vi "Dashboard Main.vi"() -> ()   [LabVIEW 2018]
uses:
  <vilib>/Utility/miscctls.llb/LVRowAndColumnTypeDef.ctl
  <vilib>/event_ctls.llb/eventvkey.ctl
  <vilib>/Rock Robotics/Network Tables/NT Read Boolean.vi
  <vilib>/Rock Robotics/WPI/Dashboard/WPI_DashboardLogging Global.vi
panel:
  in  "Camera Settings Right":T1={"Frame Rate"=30, "Compression"=30, "Size"=1, "DB Camera Config"=FALSE} {"Frame Rate" scale=1.0..30.0; "Compression" scale=100.0..-1.0; "Size" items=["640x480", "320x240", "160x120"]}
  in  "Camera Name Right":string(combo)="No Camera Selection"
  out "Camera Perf":string
  in  "Camera Settings":T1={"Frame Rate"=30, "Compression"=30, "Size"=1, "DB Camera Config"=FALSE} {"Frame Rate" scale=1.0..30.0; "Compression" scale=100.0..-1.0; "Size" items=["640x480", "320x240", "160x120"]}
  in  "TCP":refnum<k5>
  in  "Rec Mode":enum32{"Stop", "Record", "Playback"}(radio)
  out "Robot IP":string
  out "Image Message":string="Timeout in Camera Communications"
  in  "Dashboard Tab":T2(tab)
  out "Total":bool
  out "Total":dbl(slide) scale=0.0..150.0
  out "Intake":bool
  out "Intake":dbl(slide) scale=0.0..30.0
  out "B2":bool
  out "B1":bool
  out "B2":dbl(slide) scale=0.0..40.0
  out "B1":dbl(slide) scale=0.0..40.0
  out "EL2":bool
  out "EL1":bool
  out "EL2":dbl(slide) scale=0.0..40.0
  out "EL1":dbl(slide) scale=0.0..40.0
  out "BR":bool
  out "BL":bool
  out "FR":bool
  out "FL":bool
  out "BR":dbl(slide) scale=0.0..40.0
  out "BL":dbl(slide) scale=0.0..40.0
  out "FR":dbl(slide) scale=0.0..40.0
  out "FL":dbl(slide) scale=0.0..40.0
  in  "Select Auto":string(combo)="Select Autonomous ..."
  out "NT Connection":bool
  out "Gyro":dbl(knob) scale=0.0..360.0
  out "JS1 Z":dbl(slide) scale=-1.0..1.0 scale format="%#_2e"
  out "JS1 Graph":cluster{"X":dbl, "Y":dbl}[](graph)
  out "JS1 Buttons":T3
  out "JS2 Z":dbl(slide) scale=-1.0..1.0 scale format="%#_2e"
  out "JS2 Graph":cluster{"X":dbl, "Y":dbl}[](graph)
  out "JS2 Buttons":T3
  out "Mode":T4(ring)=enum."Auto Disabled"
  out "Right Camera Perf":cluster{"Bandwidth (Mbps)":dbl, "FPS":dbl}
  out "Camera Image Right":T5(plugin-control)
  in  "DB/String 9":string
  in  "DB/String 8":string
  in  "DB/String 7":string
  in  "DB/String 6":string
  in  "DB/String 5":string
  in  "DB/String 4":string
  in  "DB/String 3":string
  in  "DB/String 2":string
  in  "DB/String 1":string
  in  "DB/String 0":string
  in  "DB/Slider 0":dbl(slide) scale=0.0..5.0
  in  "DB/Slider 1":dbl(slide) scale=0.0..5.0
  in  "DB/Slider 2":dbl(slide) scale=0.0..5.0
  in  "DB/Slider 3":dbl(slide) scale=0.0..5.0
  out "DB/LED 3":bool
  out "DB/LED 2":bool
  out "DB/LED 1":bool
  out "DB/LED 0":bool
  in  "DB/Button 3":bool
  in  "DB/Button 2":bool
  in  "DB/Button 1":bool
  in  "DB/Button 0":bool caption="New Name"
  in  "Test Slider":dbl(slide) scale=0.0..100.0 scale format="%#_3g"
  in  "On/Off":bool caption="Solenoid"
  in  "Test Name":u16(ring) items=["Select the test to run..."]
  in  "Test Tree":string(tree)
  in  "Motor":cluster{"Value":dbl, "Enable":bool} {"Value" scale=-1.0..1.0 scale format="%#_3g"}
  out "Progress":T6 {"Test Progress" scale=0.0..100.0}
  in  "Rev/Fwd":cluster{"Forward":bool, "Reverse":bool}
  in  "Test Ring":u16(ring) items=["Monochrome", "Color"]
  out "Cmd Status":string
  in  "Execute Command":bool
  in  "Command Params":string[][](table)
  in  "Command Selection":i32(listbox)
  in  "CheckList":i32(listbox)
  out "Tree":string(tree)
  out "Camera Image":T5(plugin-control)
  out "Background":bool
  in  "Camera Name":string(combo)="No Camera Selection"
  # "HW"
  # "HW"
  # "Joysticks"
  # "Drive Motors"
  # "Elevator"
  # "Four Bar"
  # "Intake"
  # "Total"
  # "This tab is a great place for autonomous settings and robot-specific values.\nPlace controls and indicators inside this tab and match name to\nDashboard Variables on robot. You can also delete this comment."
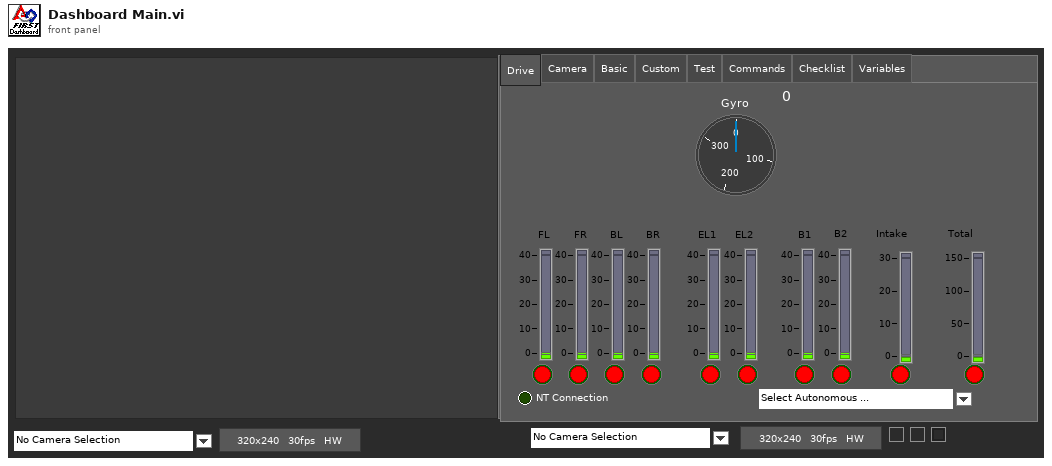
[diagram p1: front panel]
types:
  T1 = cluster{"Frame Rate":i32, "Compression":i32, "Size":u16, "DB Camera Config":bool}
  T2 = enum32{"Drive", "Camera", "Basic", "Custom", "Test", "Commands", "Checklist", "Variables"}
  T3 = cluster{bool, bool, bool, bool, bool, bool, bool, bool, bool, bool, bool, bool}
  T4 = enum8{"Tele-Op Disabled", "Tele-Op Enabled", "Auto Disabled", "Auto Enabled", "Test Disabled", "Test Enabled", "Disconnected", "No Code", "E-Stop"}
  T5 = typedef "IMAQ Image.ctl" = refnum<image>
  T6 = cluster{"Test Progress":u8, "Test Progress Text":string}
  T7 = cluster{"Save Path":path, "Interval (s)":dbl, "Keep":i32}
  T8 = typedef "Image Type" = u32
  T9 = cluster{"IDs":cluster{"RPC field ID":u16, "Unique ID":u16}, "String":string}
  T10 = cluster{"Error Strings":string, "Disable Counts":cluster{u16, u16}, "Rail Faults":cluster{u16, u16, u16}, "Robot IP":string, "DB Mode":u8, "Event Info":cluster{"Name":string, "Type":u8, "Number":u16, "Replay":u8}}
  T11 = cluster{"Storage":cluster{"Disk Free":u64, "RAM Block":u32, "RAM free":u32}, "CPU Utilization":cluster{"CPU % ISR":sgl, "CPU % Time Crit":sgl, "CPU % Timed Str":sgl, "CPU % High":sgl, "CPU % Above":sgl, "CPU % Normal":sgl, "CPU % Low":sgl}, "CAN":cluster{"% Bus Utilization":sgl, "Bus Off Cnt":u32, "TX_FIFO Full Cnt":u32, "Receive Error Cnt":u8, "Transmit Error Cnt":u8}, "HID":cluster{"HID Outputs":u32, "Rumble Low":u16, "Rumble High":u16}[]}
  T12 = cluster{"Status bits":cluster{"Test Mode":bool, "Autonomous":bool, "Enabled":bool, "Code Start":bool, "Brownout":bool, "Reserved 2":bool, "Reserved 3":bool, "E-Stop":bool}, "Code Trace":cluster{"Disabled":bool, "TeleOp":bool, "Auto":bool, "Test":bool}, "Controller Type":enum16{"unknown", "cRIO", "roboRio"}, "Code?":enum16{"unknown", "noCode", "code"}, "Battery V":dbl}
  T13 = cluster{"Control Bits":cluster{"TestMode":bool, "Autonomous":bool, "Enabled":bool, "FMS Present":bool, bool, bool, bool, "E-Stop":bool}, "Team Station ":u8, "Countdown":sgl, "Joystick Values":cluster{"Axes":dbl[], "Buttons":bool[], "POVs":i16[]}[]}
  T14 = cluster{"Axes":dbl[], "Buttons":bool[], "POVs":i16[]}[]
  T15 = cluster{"Axes":dbl[], "Buttons":bool[], "POVs":i16[]}
  T16 = cluster{"Buttons[0]":bool, "Buttons[1]":bool, "Buttons[2]":bool, "Buttons[3]":bool, "Buttons[4]":bool, "Buttons[5]":bool, "Buttons[6]":bool, "Buttons[7]":bool, "Buttons[8]":bool, "Buttons[9]":bool, "Buttons[10]":bool, "Buttons[11]":bool}
  T17 = cluster{"Camera Image":refnum<vi>, "Dashboard Tab":refnum<vi>, "Background":refnum<vi>, "Rec Mode":refnum<vi>, "Test Slider":refnum<vi>, "On/Off ":refnum<vi>, "Test Ring":refnum<vi>, "Rev/Fwd":refnum<vi>, "Test Name":refnum<vi>, "Motor":refnum<vi>, "Progress":refnum<vi>, "CheckList":refnum<vi>, "Tree":refnum<vi>, "Test Tree":refnum<vi>, "Command Params":refnum<vi>, "Command Selection":refnum<vi>, "Execute Command":refnum<vi>, "Cmd Status":refnum<vi>, "Camera Settings":refnum<vi>, "Camera Name":refnum<vi>, "Camera Perf":refnum<vi>, "Camera Settings Right":refnum<vi>, "Camera Name Right":refnum<vi>, "Camera Image Right":refnum<vi>}
  T18 = cluster{"Global Rectangle":i32[], "Contours":cluster{"Contour Type":u32, "ROI Type":u32, "Points":i32[]}[]}
  T19 = cluster{"Camera Name":string, string, "Saved DB Images Info":cluster{"Save Path":path, "Interval (s)":dbl, "Keep":i32}}
  T20 = cluster{"Camera Name Right":string, string, "Saved DB Images Info":cluster{"Save Path":path, "Interval (s)":dbl, "Keep":i32}}
  T21 = cluster{"Operation":enum16{"Update", "Clear"}, "Color Box":u32}[]
  T22 = typedef "eventvkey.ctl" = enum16{"ASCII", "Enter", "Return", "Shift", "Ctrl", "Alt", "Cmd", "Opt", "Caps", "NumLock", "Clear", "Break", "Up", "Down", "Left", "Right", "Insert", "Delete", "Home", "End", "PageUp", "PageDown", "Escape", "Help", "Pause", "ScrollLock", "F1", "F2", "F3", "F4", "F5", "F6", "F7", "F8", "F9", "F10", "F11", "F12", "F13", "F14", "F15", "F16", "F17", "F18", "F19", "F20", "F21", "F22", "F23", "F24", "Play", "VolumeUp", "VolumeDown", "Mute", "Two Byte Char"}
  T23 = cluster{"Image Size":bool, "Image Type":bool, "Pixel Value":bool, "ROI Information":bool, "Zoom Factor":bool}
  T24 = cluster{"Operation":enum16{"Update", "Clear"}, "Color Box":u32}
  T25 = typedef "LVRowAndColumnTypeDef.ctl" = cluster{"Row":i32, "Column":i32}
  T26 = cluster{"Shift":bool, "Ctrl":bool, "Alt":bool, "Cmd":bool, "Opt":bool}
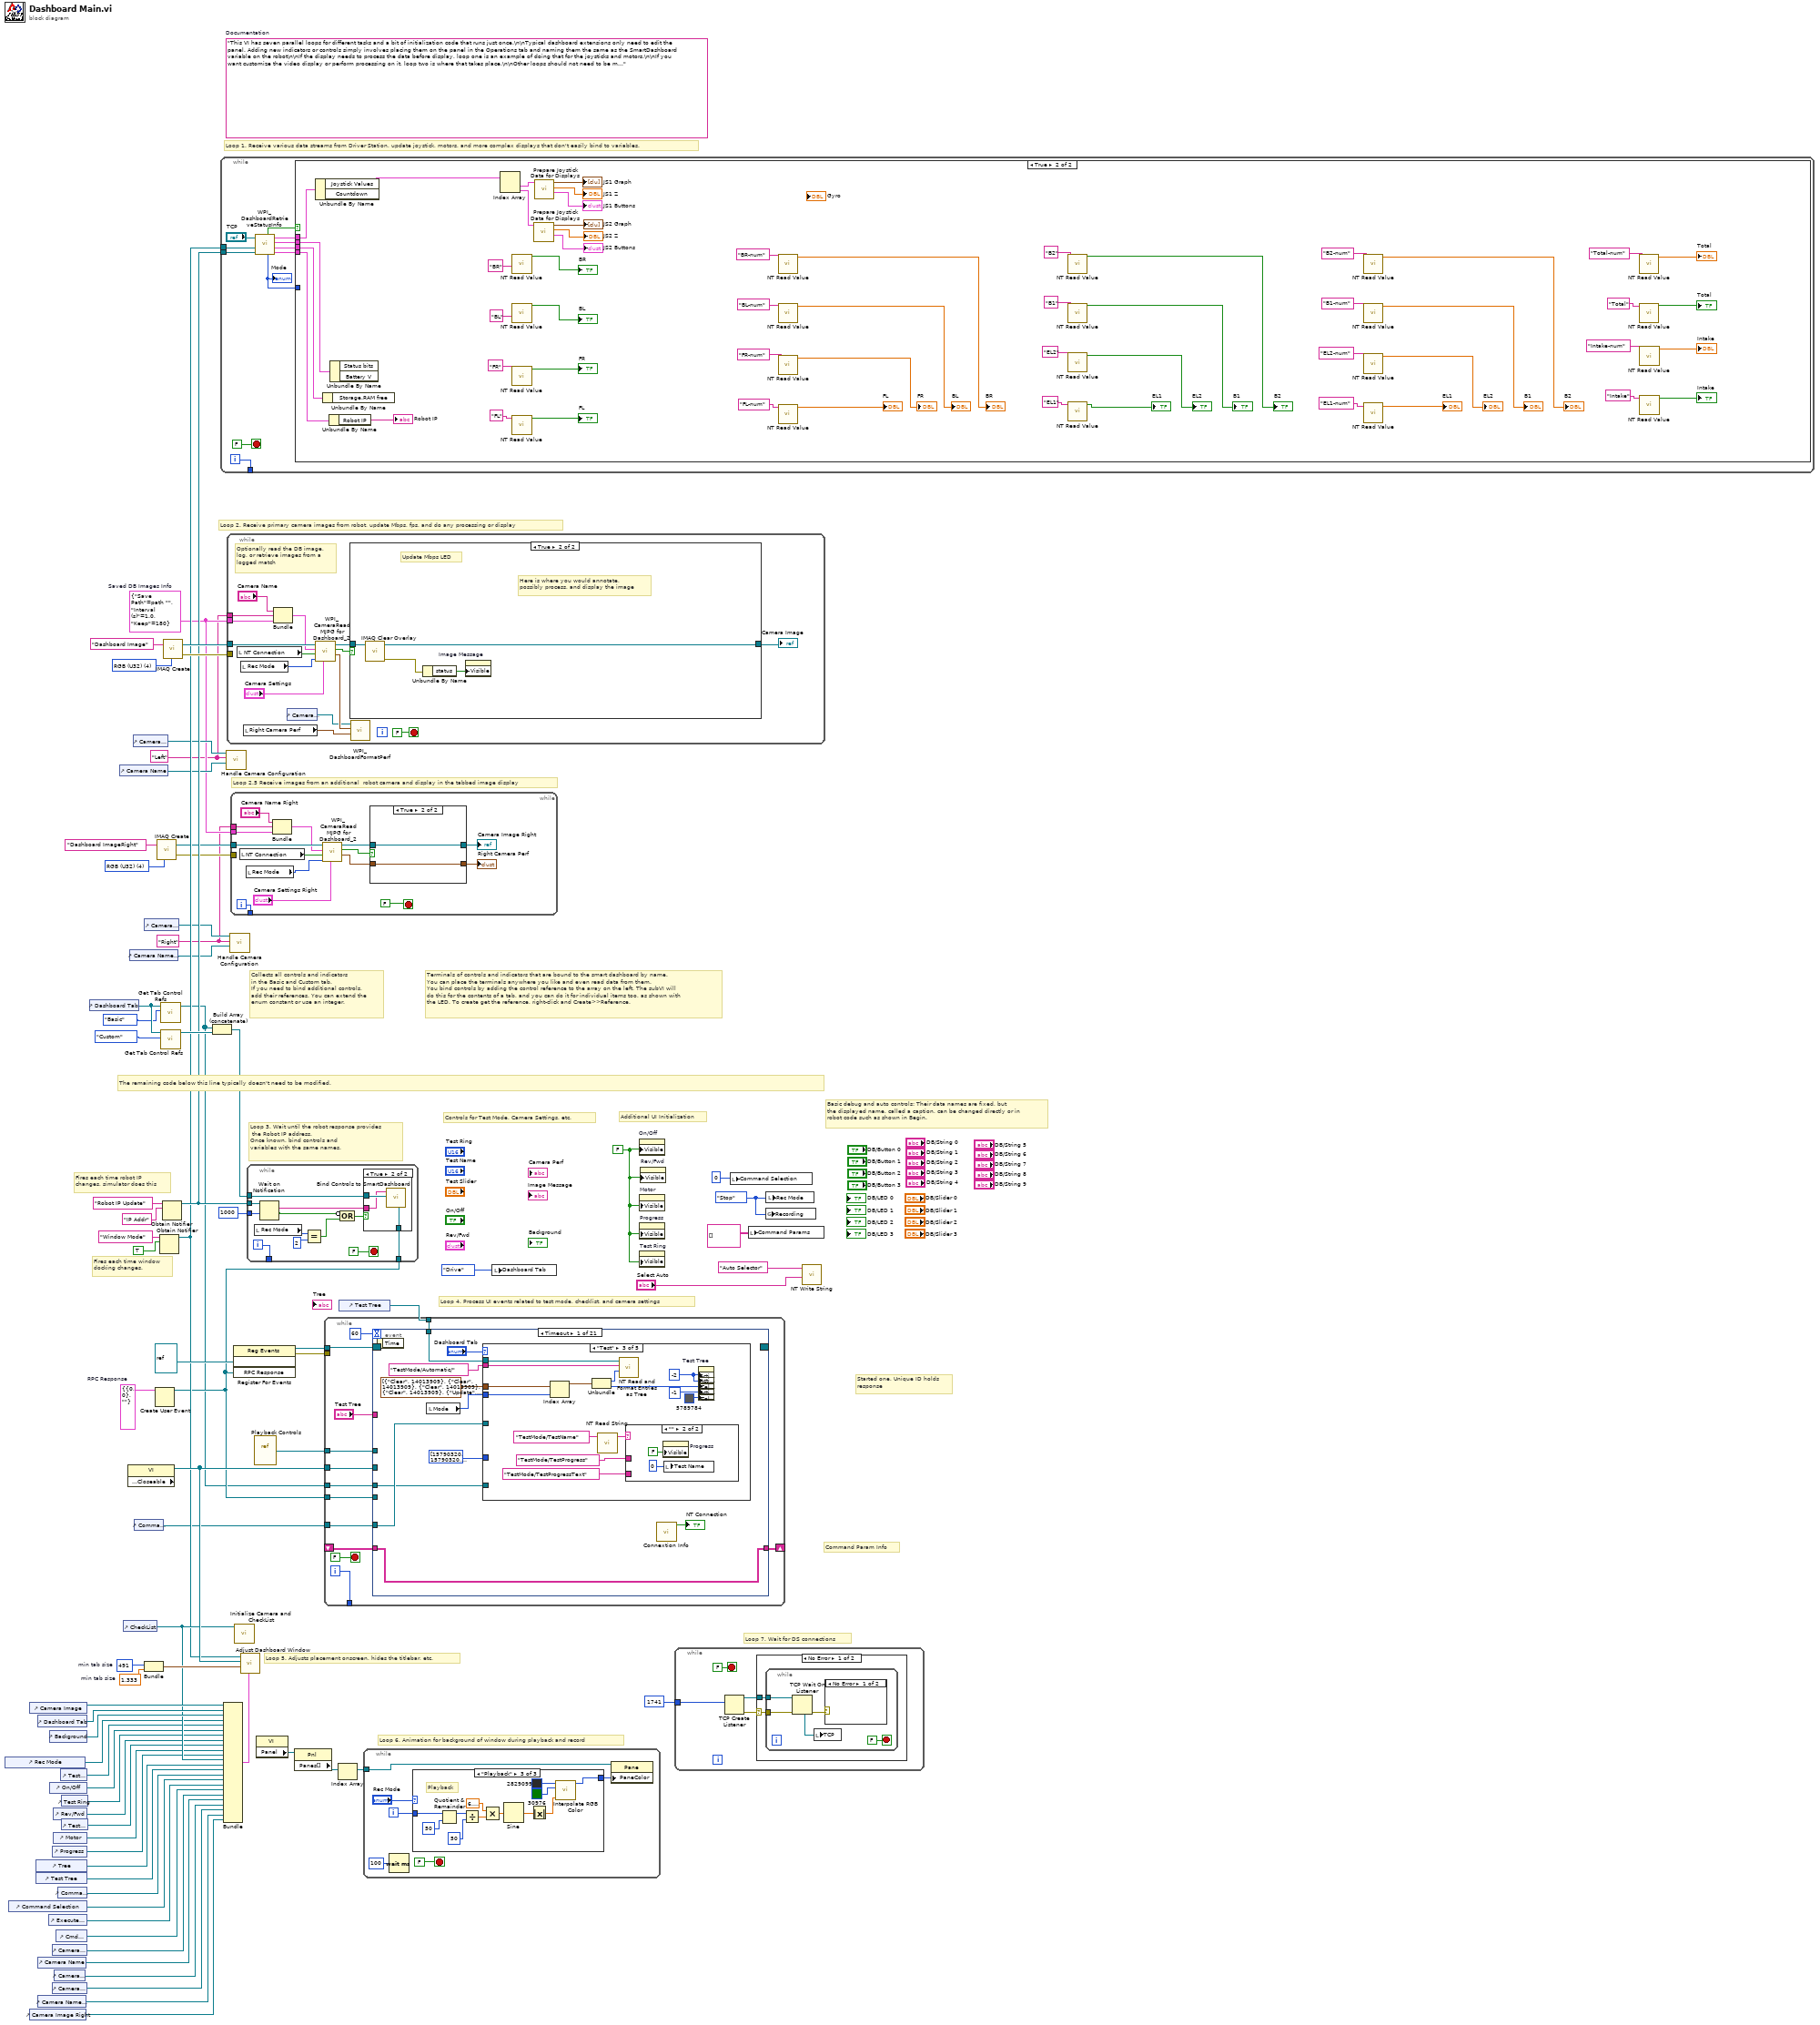
[diagram p0: block diagram]
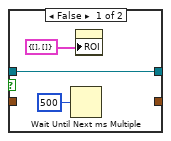
[diagram p2: hidden frame]
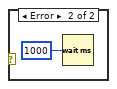
[diagram p3: hidden frame]
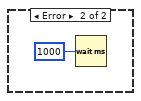
[diagram p4: hidden frame]
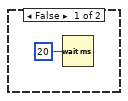
[diagram p5: hidden frame]
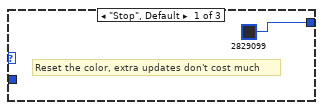
[diagram p6: hidden frame]
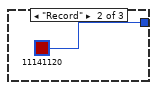
[diagram p7: hidden frame]
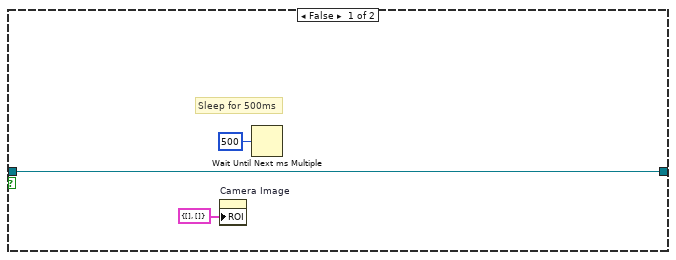
[diagram p9: hidden frame]
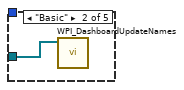
[diagram p11: hidden frame]
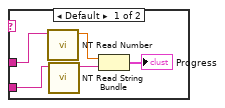
[diagram p12: hidden frame]
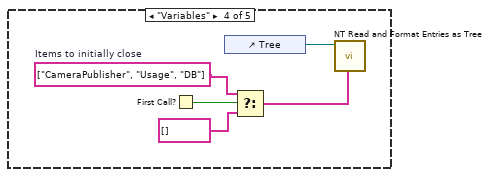
[diagram p13: hidden frame]
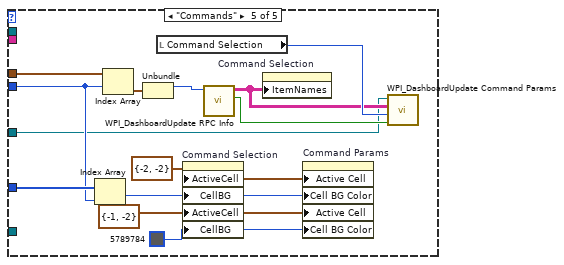
[diagram p14: hidden frame]
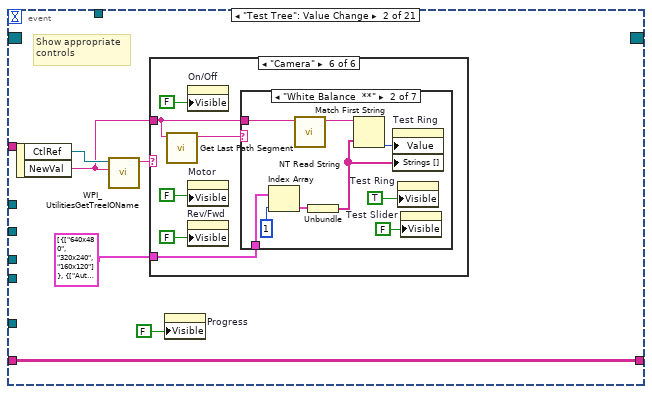
[diagram p15: hidden frame]
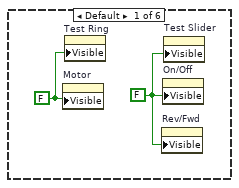
[diagram p16: hidden frame]
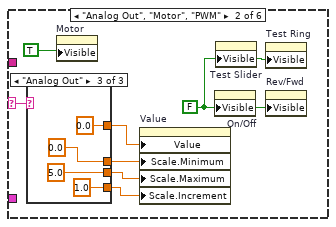
[diagram p17: hidden frame]
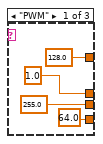
[diagram p18: hidden frame]
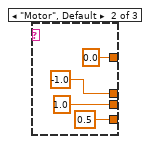
[diagram p19: hidden frame]
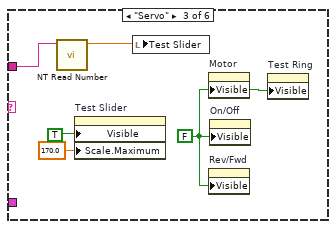
[diagram p20: hidden frame]
diagram:
  w3 = T7 {"Save Path"=path "", "Interval (s)"=1.0, "Keep"=180}  # Saved DB Images Info
  w2 = "Right"
  w1 = "Left"
  w13 = T8 4 items=["Grayscale (U8)", "Grayscale (I16)", "Grayscale (SGL)", "Complex (CSG)", "RGB (U32)", "HSL (U32)", "RGB (U64)"] ("Image Type")
  w29 = T9 {"IDs"={"RPC field ID"=0, "Unique ID"=0}, "String"=""}  # RPC Response
  w52 = 491  # min tab size
  w51 = 1.333  # min tab size
  w59 = enum32{"Stop", "Record", "Playback"}."Stop" ("Rec Mode")
  w36 = FALSE ("Visible")
  (unwired) "This VI has seven parallel loops for different tasks and a bit of initialization code that runs just once.\n\nTypical dashboard extensions only need to edit the panel. Adding new indicators or controls simply involves placing them on the panel in the Operations tab and naming them the same as the SmartDashboard variable on the robot\n\nIf the display needs to process the data before display, loop one is an example of doing that for the joysticks and motors.\n\nIf you want customize the video display or perform processing on it, loop two is where that takes place.\n\nOther loops should not need to be modified. They are pretty standard, and document the task they perform."  # Documentation
  w76 = T8 4 items=["Grayscale (U8)", "Grayscale (I16)", "Grayscale (SGL)", "Complex (CSG)", "RGB (U32)", "HSL (U32)", "RGB (U64)"] ("Image Type")
  # "Loop 2.5 Receive images from an additional  robot camera and display in the tabbed image display"
  # "Command Param Info"
  # "Started one, Unique ID holds\nresponse"
  # "Loop 7. Wait for DS connections"
  # "Basic debug and auto controls: Their data names are fixed, but\nthe displayed name, called a caption, can be changed directly or in\nrobot code such as shown in Begin."
  # "Controls for Test Mode, Camera Settings, etc."
  # "Additional UI Initialization"
  # "Loop 6. Animation for background of window during playback and record"
  # "Fires each time robot IP\nchanges, simulator does this"
  # "Fires each time window\ndocking changes."
  # "Collects all controls and indicators\nin the Basic and Custom tab.\nIf you need to bind additional controls,\nadd their references. You can extend the\nenum constant or use an integer."
  # "The remaining code below this line typically doesn't need to be modified."
  # "Loop 4. Process UI events related to test mode, checklist, and camera settings"
  # "Terminals of controls and indicators that are bound to the smart dashboard by name.\nYou can place the terminals anywhere you like and even read data from them.\nYou bind controls by adding the control reference to the array on the left. The subVI will\ndo this for the contents of a tab, and you can do it for individual items too, as shown with\nthe LED. To create get the reference, right-click and Create>>Reference."
  # "Loop 3. Wait until the robot response provides\n the Robot IP address.\nOnce known, bind controls and\nvariables with the same names."
  # "Loop 5. Adjusts placement onscreen, hides the titlebar, etc."
  # "Loop 1. Receive various data streams from Driver Station, update joystick, motors, and more complex displays that don't easily bind to variables."
  # "Loop 2. Receive primary camera images from robot, update Mbps, fps, and do any processing or display"
  n1 = control-ref of="Rec Mode"() -> (w42:refnum<vi>)
  n2 = control-ref of="Command Selection"() -> (w28:refnum<vi>)
  n3 = control-ref of="Camera Image Right"() -> (w6:refnum<vi>)
  n4 = control-ref of="Camera Image"() -> (w54:refnum<vi>)
  n5 = control-ref of="Tree"() -> (w46:refnum<vi>)
  n6 = control-ref of="Test Tree"() -> (w45:refnum<vi>)
  n7 = control-ref of="Dashboard Tab"() -> (w53:refnum<vi>)
  n8 = control-ref of="Camera Name"() -> (w19:refnum<vi>)
  n9 = control-ref of="Camera Name Right"() -> (w7:refnum<vi>)
  n10 = control-ref of="Execute Command"() -> (w30:refnum<vi>)
  n11 = control-ref of="Background"() -> (w49:refnum<vi>)
  n12 = control-ref of="On/Off"() -> (w40:refnum<vi>)
  n13 = control-ref of="Progress"() -> (w37:refnum<vi>)
  n14 = control-ref of="Camera Settings"() -> (w20:refnum<vi>)
  n15 = control-ref of="Camera Settings Right"() -> (w8:refnum<vi>)
  n16 = control-ref of="Rev/Fwd"() -> (w38:refnum<vi>)
  n17 = control-ref of="Motor"() -> (w43:refnum<vi>)
  n18 = control-ref of="Camera Perf"() -> (w18:refnum<vi>)
  n19 = control-ref of="Cmd Status"() -> (w24:refnum<vi>)
  n20 = control-ref of="Command Params"() -> (w31:refnum<vi>)
  n21 = control-ref of="Test Slider"() -> (w41:refnum<vi>)
  n22 = control-ref of="Test Ring"() -> (w39:refnum<vi>)
  n23 = control-ref of="Test Name"() -> (w44:refnum<vi>)
  n24 = control-ref of="Dashboard Tab"() -> (w57:refnum<vi>)
  n25 = control-ref of="Camera Name"() -> (w21:refnum<vi>)
  n26 = control-ref of="CheckList"() -> (w47:refnum<vi>)
  n27 = property class="VI" props=["Front Panel.Closeable"]() -> (reference out=w58:refnum<vi>)  [unwired: 2 in, 2 out]
  n28 = control-ref of="Camera Name Right"() -> (w9:refnum<vi>)
  n29 = control-ref of="Camera Settings"() -> (w22:refnum<vi>)
  n30 = control-ref of="Command Params"() -> (w23:refnum<vi>)
  n31 = control-ref of="Camera Settings Right"() -> (w10:refnum<vi>)
  n32 = Bundle("min tab size"=w52, "min tab size"=w51) -> (w50:cluster{"min tab size":i32, "min tab size":dbl})  [unwired: 1 in]
  n33 = Create User Event(user event datatype=w29) -> (user event=w25:refnum<user-event>)  [unwired: 1 in, 1 out]
  n34 = call "IMAQ Create"("Image Name"="Dashboard ImageRight", "Image Type"=w13) -> ("New Image"=w12:T5, "error out"=w11:errorcluster)  [unwired: 2 in, 1 out]
  n35 = Obtain Notifier(name (unnamed)="Window Mode", notification data type=TRUE) -> (notifier out=w34:refnum<notifier>)  [unwired: 2 in, 2 out]
  n36 = call <vilib>:"Get Tab Control Refs.vi"("Page Index"=T2."Basic" ("Dashboard Tab"), "TabControl in"=w57) -> ("ControlsOnPage"=w17:refnum<vi>[])  [unwired: 9 in]
  n37 = call <vilib>:"Get Tab Control Refs.vi"("Page Index"=T2."Custom" ("Dashboard Tab"), "TabControl in"=w57) -> ("ControlsOnPage"=w56:refnum<vi>[])  [unwired: 9 in]
  n38 = Obtain Notifier(name (unnamed)="Robot IP Update", notification data type="IP Addr" ("name (unnamed)")) -> (notifier out=w35:refnum<notifier>)  [unwired: 2 in, 2 out]
  n39 = call "IMAQ Create"("Image Name"="Dashboard Image", "Image Type"=w76) -> ("New Image"=w74:T5, "error out"=w73:errorcluster)  [unwired: 2 in, 1 out]
  n40 = Build Array (concatenate)(w17, w56) -> (w55:refnum<vi>[])
  n41 = while {
    tunnel: [w86] -> _
    tunnel: w35 -> [w80]
    tunnel: w34 -> [w77]
    i -> [w86]
    stop <- FALSE stop-if-true
    n42 = call <vilib>:"WPI_DashboardRetrieveStatusInfo.vi"("Binding Refnum"=w80, "Window Mode Notifier"=w77, "TCP Cnx"="TCP") -> ("Power and Errors"=w81:T10, "Robot Metrics"=w84:T11, "Status Info"=w85:T12, "Control Info"=w82:T13, "Robot Mode"=w79:T4, "Process?"=w83:bool)  [unwired: 3 in]
    "Mode" <- w79
    n43 = case shown="True" w83 {
      tunnel: w85 -> [_ w142]
      tunnel: w84 -> [_ w141]
      tunnel: w82 -> [_ w140]
      tunnel: w81 -> [_ w139]
      tunnel: w79 -> [_ _]
      frame False {
        n44 = Wait (ms)(milliseconds to wait=u32 20) -> ()  [unwired: 1 out]
      }
      frame True {
        n45 = Unbundle By Name(w140) -> ("Joystick Values"=w138:T14)  [unwired: 1 out]
        n46 = Unbundle By Name(w141) -> ()  [unwired: 1 out]
        n47 = Unbundle By Name(w139) -> ("Robot IP"=→"Robot IP":string)
        n48 = Unbundle By Name(w142) -> ()  [unwired: 2 out]
        n49 = Index Array(array=w138) -> (element #1=w137:T15, element #2=w133:T15)  [unwired: 2 in]
        n50 = call-poly <vilib>:"NT Read Value.vi"("Name"="BR") -> ("Boolean"=→"BR":bool)  [unwired: 9 in, 1 out]
        n51 = call-poly <vilib>:"NT Read Value.vi"("Name"="BL") -> ("Boolean"=→"BL":bool)  [unwired: 9 in, 1 out]
        n52 = call-poly <vilib>:"NT Read Value.vi"("Name"="FR") -> ("Boolean"=→"FR":bool)  [unwired: 9 in, 1 out]
        n53 = call-poly <vilib>:"NT Read Value.vi"("Name"="FL") -> ("Boolean"=→"FL":bool)  [unwired: 9 in, 1 out]
        n54 = call "Prepare Joystick Data for Displays.vi"("Joystick Values"=w133) -> ("Buttons"=→"JS2 Buttons":T16, "Z Axis"=→"JS2 Z":dbl, "Cartesian Data"=→"JS2 Graph":cluster{"X axis":dbl, "X axis":dbl}[])  [unwired: 8 in]
        n55 = call "Prepare Joystick Data for Displays.vi"("Joystick Values"=w137) -> ("Buttons"=→"JS1 Buttons":T16, "Z Axis"=→"JS1 Z":dbl, "Cartesian Data"=→"JS1 Graph":cluster{"X axis":dbl, "X axis":dbl}[])  [unwired: 8 in]
        n56 = call-poly <vilib>:"NT Read Value.vi"("Name"="BR-num") -> ("Numeric"=→"BR":dbl)  [unwired: 9 in, 1 out]
        n57 = call-poly <vilib>:"NT Read Value.vi"("Name"="BL-num") -> ("Numeric"=→"BL":dbl)  [unwired: 9 in, 1 out]
        n58 = call-poly <vilib>:"NT Read Value.vi"("Name"="FR-num") -> ("Numeric"=→"FR":dbl)  [unwired: 9 in, 1 out]
        n59 = call-poly <vilib>:"NT Read Value.vi"("Name"="FL-num") -> ("Numeric"=→"FL":dbl)  [unwired: 9 in, 1 out]
        n60 = call-poly <vilib>:"NT Read Value.vi"("Name"="B2") -> ("Boolean"=→"B2":bool)  [unwired: 9 in, 1 out]
        n61 = call-poly <vilib>:"NT Read Value.vi"("Name"="B1") -> ("Boolean"=→"B1":bool)  [unwired: 9 in, 1 out]
        n62 = call-poly <vilib>:"NT Read Value.vi"("Name"="EL2") -> ("Boolean"=→"EL2":bool)  [unwired: 9 in, 1 out]
        n63 = call-poly <vilib>:"NT Read Value.vi"("Name"="EL1") -> ("Boolean"=→"EL1":bool)  [unwired: 9 in, 1 out]
        n64 = call-poly <vilib>:"NT Read Value.vi"("Name"="B2-num") -> ("Numeric"=→"B2":dbl)  [unwired: 9 in, 1 out]
        n65 = call-poly <vilib>:"NT Read Value.vi"("Name"="B1-num") -> ("Numeric"=→"B1":dbl)  [unwired: 9 in, 1 out]
        n66 = call-poly <vilib>:"NT Read Value.vi"("Name"="EL2-num") -> ("Numeric"=→"EL2":dbl)  [unwired: 9 in, 1 out]
        n67 = call-poly <vilib>:"NT Read Value.vi"("Name"="EL1-num") -> ("Numeric"=→"EL1":dbl)  [unwired: 9 in, 1 out]
        n68 = call-poly <vilib>:"NT Read Value.vi"("Name"="Total-num") -> ("Numeric"=→"Total":dbl)  [unwired: 9 in, 1 out]
        n69 = call-poly <vilib>:"NT Read Value.vi"("Name"="Total") -> ("Boolean"=→"Total":bool)  [unwired: 9 in, 1 out]
        n70 = call-poly <vilib>:"NT Read Value.vi"("Name"="Intake-num") -> ("Numeric"=→"Intake":dbl)  [unwired: 9 in, 1 out]
        n71 = call-poly <vilib>:"NT Read Value.vi"("Name"="Intake") -> ("Boolean"=→"Intake":bool)  [unwired: 9 in, 1 out]
      }
    }
  }
  n72 = Bundle("Camera Image"=w54, "Dashboard Tab"=w53, "Background"=w49, "Rec Mode"=w42, "Test Slider"=w41, "On/Off"=w40, "Test Ring"=w39, "Rev/Fwd"=w38, "Test Name"=w44, "Motor"=w43, "Progress"=w37, "CheckList"=w47, "Tree"=w46, "Test Tree"=w45, "Command Params"=w31, "Command Selection"=w28, "Execute Command"=w30, "Cmd Status"=w24, "Camera Settings"=w20, "Camera Name"=w19, "Camera Perf"=w18, "Camera Settings Right"=w8, "Camera Name Right"=w7, "Camera Image Right"=w6) -> (w48:T17)  [unwired: 1 in]
  n73 = call "Handle Camera Configuration.vi"("CameraNameRef"=w21, "Display Name"=w1, "ClusterRef"=w22) -> ()  [unwired: 9 in]
  n74 = while {
    tunnel: w74 -> [w156]
    tunnel: w73 -> [_]
    tunnel: w3 -> [w149]
    tunnel: w1 -> [w146]
    stop <- FALSE stop-if-true
    # "Optionally read the DB image,\nlog, or retrieve images from a\nlogged match"
    n75 = local read "NT Connection"() -> (w150:bool)
    n76 = local read "Rec Mode"() -> (w153:enum32{"Stop", "Record", "Playback"})
    n77 = local read "Right Camera Perf"() -> (w144:cluster{"Bandwidth (Mbps)":dbl, "FPS":dbl})
    n78 = Bundle("Camera Name"="Camera Name", w146, "Saved DB Images Info"=w149) -> (w148:T19)  [unwired: 1 in]
    n79 = control-ref of="Camera Perf"() -> (w143:refnum<vi>)
    n80 = call <vilib>:"WPI_CameraRead MJPG for Dashboard_2.vi"("Camera Settings"="Camera Settings", "Rec Mode"=w153, "NT Connection"=w150, "Capture Info"=w148, "Image in"=w156) -> ("perf info"=w145:cluster{"Bandwidth (Mbps)":dbl, "fps":dbl}, "Active"=w154:bool, "Image\\ out"=w155:T5)  [unwired: 4 in]
    n81 = case shown="True" w154 {
      tunnel: w155 -> [w159 w162]
      tunnel: [w159 w161] -> w151
      frame False {
        # "Sleep for 500ms"
        n82 = property on="Camera Image" class="ImageControl"("ROI"=T18 {"Global Rectangle"=[], "Contours"=[]}) -> ()  [unwired: 2 in, 2 out]
        n83 = Wait Until Next ms Multiple(millisecond multiple=u32 500) -> ()  [unwired: 1 out]
      }
      frame True {
        # "Here is where you would annotate,\npossibly process, and display the image"
        # "Update Mbps LED"
        n84 = call "IMAQ Clear Overlay"("Image"=w162) -> ("error out"=w163:errorcluster, "Image Out"=w161:T5)  [unwired: 2 in, 7 out]
        n85 = Unbundle By Name(w163) -> ("status"=w164:bool)
        n86 = property on="Image Message" class="Str"("Visible"=w164) -> ()  [unwired: 2 in, 2 out]
      }
    }
    "Camera Image" <- w151
    n87 = call <vilib>:"WPI_DashboardFormatPerf.vi"("Right Camera Perf"=w144, "Performance"=w145, "String in"=w143) -> ()  [unwired: 9 in]
  }
  n88 = call "Handle Camera Configuration.vi"("CameraNameRef"=w9, "Display Name"=w2, "ClusterRef"=w10) -> ()  [unwired: 9 in]
  n89 = while {
    tunnel: w12 -> [w179]
    tunnel: w11 -> [_]
    tunnel: [w174] -> _
    tunnel: w3 -> [w170]
    tunnel: w2 -> [w167]
    i -> [w174]
    stop <- FALSE stop-if-true
    n90 = local read "NT Connection"() -> (w171:bool)
    n91 = local read "Rec Mode"() -> (w178:enum32{"Stop", "Record", "Playback"})
    n92 = Bundle("Camera Name Right"="Camera Name Right", w167, "Saved DB Images Info"=w170) -> (w169:T20)  [unwired: 1 in]
    n93 = call <vilib>:"WPI_CameraRead MJPG for Dashboard_2.vi"("Camera Settings"="Camera Settings Right", "Rec Mode"=w178, "NT Connection"=w171, "Capture Info"=w169, "Image in"=w179) -> ("perf info"=w165:cluster{"Bandwidth (Mbps)":dbl, "fps":dbl}, "Active"=w173:bool, "Image\\ out"=w176:T5)  [unwired: 4 in]
    n94 = case shown="True" w173 {
      tunnel: w176 -> [w181 w184]
      tunnel: [w181 w184] -> w172
      tunnel: [_ w183] -> w166
      tunnel: w165 -> [_ w183]
      frame False {
        n95 = Wait Until Next ms Multiple(millisecond multiple=u32 500) -> ()  [unwired: 1 out]
        n96 = property on="Camera Image Right" class="ImageControl"("ROI"=T18 {"Global Rectangle"=[], "Contours"=[]}) -> ()  [unwired: 2 in, 2 out]
      }
      frame True {
      }
    }
    "Camera Image Right" <- w172
    "Right Camera Perf" <- w166
  }
  n97 = register-events(refnum<vi> refnum, w25) -> (reference out=w63:refnum<event-registration>, error out=w62:errorcluster)  [unwired: 2 in]
  n98 = call "Initialize Camera and CheckList.vi"("ListBox in"=w47) -> ()  [unwired: 11 in]
  n99 = call "Adjust Dashboard Window.vi"("Sizing Refnums"=w48, "Size Constraints"=w50, "VI"=w58, "WIn Mode"=w34) -> ()  [unwired: 8 in]
  n100 = while {
    tunnel: w55 -> [w196]
    tunnel: w35 -> [w194]
    tunnel: [w192] -> _
    tunnel: u32 1000 ("milliseconds to wait") -> [w191]
    tunnel: w25 -> [w185]
    i -> [w192]
    stop <- FALSE stop-if-true
    n101 = local read "Rec Mode"() -> (w187:enum32{"Stop", "Record", "Playback"})
    n102 = Wait on Notification(notifier=w194, timeout in ms (-1)=w191) -> (notification=w193:string, timed out?=w189:bool)  [unwired: 2 in, 2 out]
    n103 = Equal?(x=w187, y=u16 2 ("Rec Mode")) -> (x = y?=w188:bool)
    n104 = Compound Arithmetic op=OR(invert w189, w188) -> (w190:bool)
    n105 = case shown="True" w190 {
      tunnel: w196 -> [_ w199]
      tunnel: w193 -> [_ w198]
      tunnel: w185 -> [_ w197]
      frame False {
      }
      frame True {
        n106 = call <vilib>:"Bind Controls to SmartDashboard.vi"("RPC ref"=w197, "Bound Control Refs"=w199, "Server IP Address"=w198) -> ()  [unwired: 9 in]
      }
    }
  }
  n107 = vi-ref "Playback Controls.vi"() -> (w64:refnum<vi>)
  n108 = property class="VI"() -> ("Panel"=w66:refnum<vi>)  [unwired: 2 in, 2 out]
  n109 = property class="Pnl"(reference=w66) -> ("Panes[]"=w67:refnum<vi>[])  [unwired: 1 in, 2 out]
  n110 = Index Array(array=w67) -> (element=w65:refnum<vi>)  [unwired: 1 in]
  n111 = control-ref of="Test Tree"() -> (w68:refnum<vi>)
  n112 = while {
    tunnel: [w209] -> _
    tunnel: w68 -> [w208]
    tunnel: w64 -> [w207]
    tunnel: w63 -> [w206]
    tunnel: w62 -> [_]
    tunnel: w58 -> [w205]
    tunnel: w25 -> [w204]
    tunnel: w23 -> [w203]
    shift-right: [w202] -> _
    shift-left: _ -> [w201]
    tunnel: w17 -> [w200]
    i -> [w209]
    stop <- FALSE stop-if-true
    n113 = event shown="[0] Timeout" {
      selector: w206 -> [_ _ _ _ _ _ _ _ _ _ _ _ _ _ _ _ _ _ _ _ _]
      dyn-events: [_ _ _ _ _ _ _ _ _ _ _ _ _ _ _ _ w469 _ _ _ _] -> _
      timeout: u32 60 ("milliseconds to wait") -> [_ _ _ _ _ _ _ _ _ _ _ _ _ _ _ _ _ _ _ _ _]
      tunnel: w208 -> [w221 _ _ _ _ _ _ _ _ _ _ _ _ _ _ _ _ _ _ _ _]
      tunnel: "Test Tree" -> [_ _ _ _ _ _ _ _ _ _ _ w436 w444 w446 w450 w458 _ _ _ _ _]
      tunnel: w207 -> [_ _ _ _ _ _ _ _ _ _ _ _ _ _ _ _ w471 _ w489 _ _]
      tunnel: w205 -> [_ _ _ _ _ _ _ _ _ _ _ _ _ _ _ _ w467 _ _ _ _]
      tunnel: w204 -> [_ _ _ _ _ _ _ _ _ _ _ _ _ _ _ _ w465 _ _ _ _]
      tunnel: w203 -> [w216 _ _ _ _ _ w387 _ _ _ _ _ _ _ _ _ _ _ _ _ _]
      tunnel: [w215 w264 w366 w371 w380 w384 w385 w394 w404 w411 w423 w435 w442 w445 w449 w457 w464 w484 w486 w490 w503] -> w202
      tunnel: w201 -> [w215 w264 w366 w371 w380 w384 w385 _ _ w411 w423 w435 w442 w445 w449 w457 w464 w484 w486 w490 w503]
      tunnel: w200 -> [w213 _ _ _ _ _ _ _ _ _ _ _ _ _ _ _ _ _ _ _ _]
      event Timeout {
        n114 = event-data() -> ()  [unwired: 1 in, 1 out]
        n115 = local read "Mode"() -> (w218:T4)
        n116 = case shown="\"Test\"" "Dashboard Tab" {
          tunnel: w221 -> [_ _ w237 _ _]
          tunnel: "TestMode/Automatic/" ("Name Pattern") -> [_ _ w236 _ _]
          tunnel: T21 [{"Operation"=enum."Clear", "Color Box"=14013909}, {"Operation"=enum."Clear", "Color Box"=14013909}, {"Operation"=enum."Clear", "Color Box"=14013909}, {"Operation"=enum."Clear", "Color Box"=14013909}, {"Operation"=enum."Update", "Color Box"=14013909}, {"Operation"=enum."Update", "Color Box"=16777215}, {"Operation"=enum."Clear", "Color Box"=14013909}, {"Operation"=enum."Clear", "Color Box"=14013909}, {"Operation"=enum."Clear", "Color Box"=14013909}] -> [_ _ w229 _ w257]
          tunnel: w218 -> [_ _ w228 _ w256]
          tunnel: u32[] [15790320, 15790320, 15790320, 15790320, 16777215, 16777215, 15790320, 15790320, 15790320] -> [_ _ _ _ w262]
          tunnel: w216 -> [_ _ _ _ w250]
          tunnel: w213 -> [_ w223 _ _ _]
          frame "Custom", Default {
          }
          frame "Basic" {
            n117 = call <vilib>:"WPI_DashboardUpdateNames.vi"("Controls on Tab"=w223) -> ()  [unwired: 11 in]
          }
          frame "Test" {
            w235 = -2 ("Active Item:Row Number")
            n118 = Index Array(array=w229, index=w228) -> (element=w230:T24)
            n119 = Unbundle(w230) -> ("Operation"=w231:enum16{"Update", "Clear"}, "Color Box"=w232:u32)
            n120 = call <vilib>:"NT Read String.vi"("Name"="TestMode/TestName") -> ("String"=w226:string)  [unwired: 9 in, 1 out]
            n121 = call <vilib>:"NT Read and Format Entries as Tree.vi"("Operation"=w231, "Name Pattern"=w236, "Tree Refnum"=w237) -> ()  [unwired: 7 in, 2 out]
            n122 = case shown="\"\"" w226 {
              tunnel: "TestMode/TestProgress" ("Name") -> [w239 _]
              tunnel: "TestMode/TestProgressText" ("Name") -> [w238 _]
              frame Default {
                n123 = call <vilib>:"NT Read Number.vi"("Name"=w239) -> ("Numeric"=w240:dbl)  [unwired: 9 in, 1 out]
                n124 = call <vilib>:"NT Read String.vi"("Name"=w238) -> ("String"=w241:string)  [unwired: 9 in, 1 out]
                n125 = Bundle("Numeric"=w240, "String"=w241) -> (→"Progress":cluster{"Numeric":dbl, "String":string})  [unwired: 1 in]
              }
              frame "" {
                n126 = property on="Progress" class="Clust (strict)"("Visible"=FALSE) -> ()  [unwired: 2 in, 2 out]
                n127 = local write "Test Name"(u16 0) -> ()
              }
            }
            n128 = property on="Test Tree" class="Tree (strict)"("Active Item Row Number"=w235, "ActiveColNum"=w235, "CellBG"=w232, "Active Item Row Number"=-1 ("Active Item:Row Number"), "CellBG"=u32 5789784 ("Color Box")) -> ()  [unwired: 2 in, 2 out]
          }
          frame "Variables" {
            w247 = string[] ["CameraPublisher", "Usage", "DB"]  # Items to initially close
            n129 = First Call?() -> (First Call?: T/F=w248:bool)
            n130 = control-ref of="Tree"() -> (w249:refnum<vi>)
            n131 = Select(t=w247, s=w248, f=string[] []) -> (s? t:f=w245:string[])
            n132 = call <vilib>:"NT Read and Format Entries as Tree.vi"("Tags to  Close"=w245, "Tree Refnum"=w249) -> ()  [unwired: 8 in, 2 out]
          }
          frame "Commands" {
            w258 = u32 5789784 ("Color Box")
            w259 = T25 {"Row"=-1, "Column"=-2} ("Active Cell:Active Cell")
            w261 = T25 {"Row"=-2, "Column"=-2} ("Active Cell:Active Cell")
            n133 = Index Array(array=w262, index=w256) -> (element=w260:u32)
            n134 = Index Array(array=w257, index=w256) -> (element=w255:T24)
            n135 = Unbundle(w255) -> ("Operation"=w254:enum16{"Update", "Clear"})  [unwired: 1 out]
            n136 = local read "Command Selection"() -> (w253:i32)
            n137 = property on="Command Selection" class="MCListbox (strict)"("ActiveCell"=w261, "CellBG"=w260, "ActiveCell"=w259, "CellBG"=w258) -> ()  [unwired: 2 in, 2 out]
            n138 = call <vilib>:"WPI_DashboardUpdate RPC Info.vi"("Operation"=w254) -> ("update"=w252:bool, "commands"=w251:string[][])  [unwired: 9 in]
            n139 = property on="Command Selection" class="MCListbox (strict)"("ItemNames"=w251) -> ()  [unwired: 2 in, 2 out]
            n140 = property on="Command Params" class="Tbl (strict)"("Active Cell"=w261, "Cell BG Color"=w260, "Active Cell"=w259, "Cell BG Color"=w258) -> ()  [unwired: 2 in, 2 out]
            n141 = call <vilib>:"WPI_DashboardUpdate Command Params.vi"("Update"=w252, "NewVal"=w253, "Commands"=w251, "Param Tbl"=w250) -> ()  [unwired: 7 in, 1 out]
          }
        }
        n142 = call <vilib>:"Connextion Info.vi"() -> ("Connected"=→"NT Connection":bool)  [unwired: 10 in, 1 out]
      }
      event "Test Tree": Value Change {
        # "Show appropriate\ncontrols"
        n143 = event-data() -> ("CtlRef"=w267:refnum<vi>, "NewVal"=w265:string)  [unwired: 1 in]
        n144 = call <vilib>:"WPI_UtilitiesGetTreeIOName.vi"("NewVal"=w265, "TreeControl in"=w267) -> ("I/O Name"=w268:string)  [unwired: 9 in]
        n145 = case shown="\"Camera\"" w268 {
          selector: w268 -> [_ w275 _ w297 w306 _]
          tunnel: w265 -> [_ _ w294 w296 _ w313]
          tunnel: cluster{string[]}[] [{["640x480", "320x240", "160x120"]}, {["Auto", "Fixed indoor", "Fixed outdoor 1", "Fixed outdoor 2", "Fixed fluorescent 1", "Fixed fluorescent 2", "Hold current"]}, {["Auto", "Flicker-free 50 Hz", "Flicker-free 60 Hz", "Hold current"]}, {["None", "Prioritize frame rate", "Prioritize image quality"]}, {["Monochrome", "Color"]}] -> [_ _ _ _ _ w312]
          frame Default {
            w270 = FALSE ("Visible")
            w269 = FALSE ("Visible")
            n146 = property on="Motor" class="Clust (strict)"("Visible"=w269) -> ()  [unwired: 2 in, 2 out]
            n147 = property on="Test Ring" class="Ring (strict)"("Visible"=w269) -> ()  [unwired: 2 in, 2 out]
            n148 = property on="Rev/Fwd" class="Clust (strict)"("Visible"=w270) -> ()  [unwired: 2 in, 2 out]
            n149 = property on="On/Off" class="Bool (strict)"("Visible"=w270) -> ()  [unwired: 2 in, 2 out]
            n150 = property on="Test Slider" class="Slide (strict)"("Visible"=w270) -> ()  [unwired: 2 in, 2 out]
          }
          frame "Analog Out", "Motor", "PWM" {
            w276 = FALSE ("Visible")
            n151 = case shown="\"Analog Out\"" w275 {
              tunnel: [1.0 ("Value") -1.0 ("Value") 0.0 ("Value")] -> w274
              tunnel: [255.0 ("Value") 1.0 ("Value") 5.0 ("Value")] -> w273
              tunnel: [128.0 ("Value") 0.0 ("Value") 0.0 ("Value")] -> w272
              tunnel: [64.0 ("Value") 0.5 ("Value") 1.0 ("Value")] -> w271
              frame "PWM" {
              }
              frame "Motor", Default {
              }
              frame "Analog Out" {
              }
            }
            n152 = property on="Motor" class="Clust (strict)"("Visible"=TRUE) -> ()  [unwired: 2 in, 2 out]
            n153 = property on="Value" class="Slide (strict)"("Value"=w272, "Scale.Minimum"=w274, "Scale.Maximum"=w273, "Scale.Increment"=w271) -> ()  [unwired: 2 in, 2 out]
            n154 = property on="On/Off" class="Bool (strict)"("Visible"=w276) -> ()  [unwired: 2 in, 2 out]
            n155 = property on="Test Slider" class="Slide (strict)"("Visible"=w276) -> ()  [unwired: 2 in, 2 out]
            n156 = property on="Test Ring" class="Ring (strict)"("Visible"=w276) -> ()  [unwired: 2 in, 2 out]
            n157 = property on="Rev/Fwd" class="Clust (strict)"("Visible"=w276) -> ()  [unwired: 2 in, 2 out]
          }
          frame "Servo" {
            w292 = FALSE ("Visible")
            n158 = call <vilib>:"NT Read Number.vi"("Name"=w294) -> ("Numeric"=w293:dbl)  [unwired: 9 in, 1 out]
            n159 = property on="Test Slider" class="Slide (strict)"("Visible"=TRUE, "Scale.Maximum"=170.0 ("Scale.Range:Maximum")) -> ()  [unwired: 2 in, 2 out]
            n160 = local write "Test Slider"(w293) -> ()
            n161 = property on="Motor" class="Clust (strict)"("Visible"=w292) -> ()  [unwired: 2 in, 2 out]
            n162 = property on="Rev/Fwd" class="Clust (strict)"("Visible"=w292) -> ()  [unwired: 2 in, 2 out]
            n163 = property on="On/Off" class="Bool (strict)"("Visible"=w292) -> ()  [unwired: 2 in, 2 out]
            n164 = property on="Test Ring" class="Ring (strict)"("Visible"=w292) -> ()  [unwired: 2 in, 2 out]
          }
          frame "Relay", "Solenoid" {
            w295 = FALSE ("Visible")
            n165 = property on="Motor" class="Clust (strict)"("Visible"=w295) -> ()  [unwired: 2 in, 2 out]
            n166 = property on="Test Slider" class="Slide (strict)"("Visible"=w295) -> ()  [unwired: 2 in, 2 out]
            n167 = Search and Replace String(input string=w296, search string="/Value  **", replace string="/Direction") -> (result string=w302:string)  [unwired: 5 in, 3 out]
            n168 = property on="Test Ring" class="Ring (strict)"("Visible"=w295) -> ()  [unwired: 2 in, 2 out]
            n169 = call <vilib>:"NT Read String.vi"("Name"=w302) -> ("String"=w300:string)  [unwired: 9 in, 1 out]
            n170 = Equal?(x="Both directions", y=w300) -> (x = y?=w298:bool)
            n171 = Not(x=w298) -> (.not. x?=w299:bool)
            n172 = property on="Rev/Fwd" class="Clust (strict)"("Visible"=w298) -> ()  [unwired: 2 in, 2 out]
            n173 = property on="On/Off" class="Bool (strict)"("Visible"=w299, "Caption.Text"=w297) -> ()  [unwired: 2 in, 2 out]
          }
          frame "Compressor", "Digital Out" {
            w305 = FALSE ("Visible")
            # "Get direction and finish"
            n174 = property on="Motor" class="Clust (strict)"("Visible"=w305) -> ()  [unwired: 2 in, 2 out]
            n175 = property on="Test Slider" class="Slide (strict)"("Visible"=w305) -> ()  [unwired: 2 in, 2 out]
            n176 = property on="Test Ring" class="Ring (strict)"("Visible"=w305) -> ()  [unwired: 2 in, 2 out]
            n177 = property on="On/Off" class="Bool (strict)"("Visible"=TRUE, "Caption.Text"=w306) -> ()  [unwired: 2 in, 2 out]
            n178 = property on="Rev/Fwd" class="Clust (strict)"("Visible"=FALSE) -> ()  [unwired: 2 in, 2 out]
          }
          frame "Camera" {
            n179 = call <vilib>:"Get Last Path Segment.vi"("String in"=w313) -> ("String out"=w314:string)  [unwired: 10 in]
            n180 = property on="On/Off" class="Bool (strict)"("Visible"=FALSE) -> ()  [unwired: 2 in, 2 out]
            n181 = property on="Motor" class="Clust (strict)"("Visible"=FALSE) -> ()  [unwired: 2 in, 2 out]
            n182 = property on="Rev/Fwd" class="Clust (strict)"("Visible"=FALSE) -> ()  [unwired: 2 in, 2 out]
            n183 = case shown="\"White Balance  **\"" w314 {
              tunnel: w313 -> [w320 w329 w338 w347 w356 _ w362]
              tunnel: w312 -> [w318 w326 w335 w344 w353 _ _]
              frame "Size  **" {
                n184 = Index Array(array=w318) -> (element=w317:cluster{string[]})  [unwired: 1 in]
                n185 = call <vilib>:"NT Read String.vi"("Name"=w320) -> ("String"=w319:string)  [unwired: 9 in, 1 out]
                n186 = Unbundle(w317) -> (w315:string[])
                n187 = Match First String(2:w315, 3:w319) -> (0:w316:i32)  [unwired: 1 out]
                n188 = property on="Test Ring" class="Ring (strict)"("Value"=w316, "Strings []"=w315) -> ()  [unwired: 2 in, 2 out]
                n189 = property on="Test Ring" class="Ring (strict)"("Visible"=TRUE) -> ()  [unwired: 2 in, 2 out]
                n190 = property on="Test Slider" class="Slide (strict)"("Visible"=FALSE) -> ()  [unwired: 2 in, 2 out]
              }
              frame "White Balance  **" {
                n191 = Index Array(array=w326, index=1) -> (element=w327:cluster{string[]})
                n192 = call <vilib>:"NT Read String.vi"("Name"=w329) -> ("String"=w328:string)  [unwired: 9 in, 1 out]
                n193 = Unbundle(w327) -> (w324:string[])
                n194 = Match First String(2:w324, 3:w328) -> (0:w323:i32)  [unwired: 1 out]
                n195 = property on="Test Ring" class="Ring (strict)"("Value"=w323, "Strings []"=w324) -> ()  [unwired: 2 in, 2 out]
                n196 = property on="Test Ring" class="Ring (strict)"("Visible"=TRUE) -> ()  [unwired: 2 in, 2 out]
                n197 = property on="Test Slider" class="Slide (strict)"("Visible"=FALSE) -> ()  [unwired: 2 in, 2 out]
              }
              frame "Exposure  **" {
                n198 = Index Array(array=w335, index=2) -> (element=w336:cluster{string[]})
                n199 = call <vilib>:"NT Read String.vi"("Name"=w338) -> ("String"=w337:string)  [unwired: 9 in, 1 out]
                n200 = Unbundle(w336) -> (w332:string[])
                n201 = Match First String(2:w332, 3:w337) -> (0:w333:i32)  [unwired: 1 out]
                n202 = property on="Test Ring" class="Ring (strict)"("Value"=w333, "Strings []"=w332) -> ()  [unwired: 2 in, 2 out]
                n203 = property on="Test Ring" class="Ring (strict)"("Visible"=TRUE) -> ()  [unwired: 2 in, 2 out]
                n204 = property on="Test Slider" class="Slide (strict)"("Visible"=FALSE) -> ()  [unwired: 2 in, 2 out]
              }
              frame "Exposure Priority  **" {
                n205 = Index Array(array=w344, index=3) -> (element=w345:cluster{string[]})
                n206 = call <vilib>:"NT Read String.vi"("Name"=w347) -> ("String"=w346:string)  [unwired: 9 in, 1 out]
                n207 = Unbundle(w345) -> (w341:string[])
                n208 = Match First String(2:w341, 3:w346) -> (0:w342:i32)  [unwired: 1 out]
                n209 = property on="Test Ring" class="Ring (strict)"("Value"=w342, "Strings []"=w341) -> ()  [unwired: 2 in, 2 out]
                n210 = property on="Test Ring" class="Ring (strict)"("Visible"=TRUE) -> ()  [unwired: 2 in, 2 out]
                n211 = property on="Test Slider" class="Slide (strict)"("Visible"=FALSE) -> ()  [unwired: 2 in, 2 out]
              }
              frame "Color Enable  **" {
                n212 = Index Array(array=w353, index=4) -> (element=w354:cluster{string[]})
                n213 = call <vilib>:"NT Read String.vi"("Name"=w356) -> ("String"=w355:string)  [unwired: 9 in, 1 out]
                n214 = Unbundle(w354) -> (w350:string[])
                n215 = Match First String(2:w350, 3:w355) -> (0:w351:i32)  [unwired: 1 out]
                n216 = property on="Test Ring" class="Ring (strict)"("Value"=w351, "Strings []"=w350) -> ()  [unwired: 2 in, 2 out]
                n217 = property on="Test Ring" class="Ring (strict)"("Visible"=TRUE) -> ()  [unwired: 2 in, 2 out]
                n218 = property on="Test Slider" class="Slide (strict)"("Visible"=FALSE) -> ()  [unwired: 2 in, 2 out]
              }
              frame Default {
                n219 = property on="Test Ring" class="Ring (strict)"("Visible"=FALSE) -> ()  [unwired: 2 in, 2 out]
                n220 = property on="Test Slider" class="Slide (strict)"("Visible"=FALSE) -> ()  [unwired: 2 in, 2 out]
              }
              frame "Brightness  **", "Color Level  **", "Compression  **", "FPS  **", "Sharpness  **" {
                n221 = call <vilib>:"NT Read Number.vi"("Name"=w362) -> ("Numeric"=w361:dbl)  [unwired: 9 in, 1 out]
                n222 = local write "Test Slider"(w361) -> ()
                n223 = property on="Test Slider" class="Slide (strict)"("Visible"=TRUE, "Scale.Maximum"=100.0 ("Scale.Range:Maximum")) -> ()  [unwired: 2 in, 2 out]
                n224 = property on="Test Ring" class="Ring (strict)"("Visible"=FALSE) -> ()  [unwired: 2 in, 2 out]
              }
            }
          }
        }
        n225 = property on="Progress" class="Clust (strict)"("Visible"=FALSE) -> ()  [unwired: 2 in, 2 out]
      }
      event "Test Name": Mouse Enter {
        # "Populate the ring with the list of tests"
        n226 = event-data() -> ()  [unwired: 1 in, 1 out]
        n227 = call <vilib>:"NT Read String Array.vi"("Name"="TestMode/TestList") -> ("String Array"=w370:string[])  [unwired: 9 in, 1 out]
        n228 = Build Array (concatenate)("Select the test to run...", w370) -> (w369:string[])
        n229 = property on="Test Name" class="Ring (strict)"("Strings []"=w369) -> ()  [unwired: 2 in, 2 out]
      }
      event "Test Name": Value Change {
        w372 = FALSE ("Visible")
        # "Tell the robot the test name to run"
        n230 = event-data() -> ("NewVal"=w376:u16)  [unwired: 1 in]
        n231 = property on="Test Name" class="Ring (strict)"() -> ("Strings []"=w377:string[])  [unwired: 2 in, 2 out]
        n232 = local write "Progress"(T6 {"Test Progress"=0, "Test Progress Text"=""} ("Progress")) -> ()
        n233 = Index Array(array=w377, index=w376) -> (element=w375:string)
        n234 = call <vilib>:"NT Write String.vi"("String"=w375, "Name"="TestMode/TestName") -> ()  [unwired: 9 in, 1 out]
        n235 = property on="Progress" class="Clust (strict)"("Visible"=TRUE) -> ()  [unwired: 2 in, 2 out]
        n236 = property on="Motor" class="Clust (strict)"("Visible"=w372) -> ()  [unwired: 2 in, 2 out]
        n237 = property on="Test Slider" class="Slide (strict)"("Visible"=w372) -> ()  [unwired: 2 in, 2 out]
        n238 = property on="On/Off" class="Bool (strict)"("Visible"=w372) -> ()  [unwired: 2 in, 2 out]
        n239 = property on="Rev/Fwd" class="Clust (strict)"("Visible"=w372) -> ()  [unwired: 2 in, 2 out]
        n240 = property on="Test Ring" class="Ring (strict)"("Visible"=w372) -> ()  [unwired: 2 in, 2 out]
      }
      event "Select Auto": Mouse Enter {
        # "Populate the combo box with the list of autonomous options"
        n241 = event-data() -> ()  [unwired: 1 in, 1 out]
        n242 = call <vilib>:"NT Read String Array.vi"("Name"="Auto List") -> ("String Array"=w379:string[])  [unwired: 9 in, 1 out]
        n243 = property on="Select Auto" class="CmbBox"("Strings[]"=w379) -> ()  [unwired: 2 in, 2 out]
      }
      event "Select Auto": Value Change {
        # "User modified the Auto Selection. Write to NT variable so robot knows."
        n244 = event-data() -> ("NewVal"=w382:string)  [unwired: 1 in]
        n245 = call <vilib>:"NT Write String.vi"("String"=w382, "Name"="Auto Selector") -> ()  [unwired: 9 in, 1 out]
      }
      event "Command Selection": Value Change {
        # "Get the params and show in table"
        n246 = event-data() -> ("NewVal"=w388:i32)  [unwired: 1 in]
        n247 = property on="Command Selection" class="MCListbox (strict)"() -> ("ItemNames"=w386:string[][])  [unwired: 2 in, 2 out]
        n248 = call <vilib>:"WPI_DashboardUpdate Command Params.vi"("NewVal"=w388, "Commands"=w386, "Param Tbl"=w387) -> ()  [unwired: 8 in, 1 out]
      }
      event "Execute Command": Value Change {
        # "Started one, Unique ID holds\nresponse"
        n249 = event-data() -> ()  [unwired: 1 in, 1 out]
        n250 = property on="Command Selection" class="MCListbox (strict)"() -> ("ItemNames"=w399:string[][])  [unwired: 2 in, 2 out]
        n251 = Index Array(array=w399, index (row)="Command Selection", index (col)=0) -> (element=w397:string)
        n252 = call <vilib>:"Invoke Commands.vi"("Command Params"="Command Params", "Function Name"=w397) -> ("Params"=w393:u8, "Started"=w392:bool)  [unwired: 7 in, 1 out]
        n253 = Array Subset(array="Command Params", length (row)=w393) -> (w394:string[][])  [unwired: 3 in]
        n254 = Select(t="Executing" ("Cmd Status"), s=w392, f="" ("Cmd Status")) -> (s? t:f=→"Cmd Status":string)
      }
      event "Command Selection": Double Click {
        n255 = event-data() -> ("Row"=w407:i32)  [unwired: 1 in]
        n256 = property on="Command Selection" class="MCListbox (strict)"() -> ("ItemNames"=w410:string[][])  [unwired: 2 in, 2 out]
        n257 = local read "Command Params"() -> (w406:string[][])
        n258 = Index Array(array=w410, index (row)=w407, index (col)=0) -> (element=w408:string)
        n259 = call <vilib>:"Invoke Commands.vi"("Command Params"=w406, "Function Name"=w408) -> ("Params"=w405:u8, "Started"=w400:bool)  [unwired: 7 in, 1 out]
        n260 = Array Subset(array=w406, length (row)=w405) -> (w404:string[][])  [unwired: 3 in]
        n261 = Select(t="Executing" ("Cmd Status"), s=w400, f="" ("Cmd Status")) -> (s? t:f=w401:string)
        n262 = local write "Cmd Status"(w401) -> ()
      }
      event "CheckList": Double Click {
        # "Shift clears all"
        # "Update symbols on the listbox"
        n263 = event-data() -> ("PlatMods.Shift"=w412:bool, "Row"=w414:i32)  [unwired: 1 in]
        n264 = case shown="True" w412 {
          tunnel: w414 -> [w418 _]
          tunnel: 1 -> [w417 _]
          frame False {
            n265 = property on="CheckList" class="LstBox (strict)"() -> ("Item Symbols"=w416:i32[])  [unwired: 2 in, 2 out]
            n266 = Replace Array Subset(array=w416, new element=w417, index=w418) -> (w415:i32[])
            n267 = property on="CheckList" class="LstBox (strict)"("Item Symbols"=w415) -> ()  [unwired: 2 in, 2 out]
          }
          frame True {
            w419 = 0 ("Top Row")
            n268 = property on="CheckList" class="LstBox (strict)"() -> ("Number of Rows"=w421:u32)  [unwired: 2 in, 2 out]
            n269 = Initialize Array(0, w421) -> (w420:i32[])
            n270 = property on="CheckList" class="LstBox (strict)"("Top Row"=w419, "Value"=w419, "Item Symbols"=w420) -> ()  [unwired: 2 in, 2 out]
          }
        }
      }
      event "CheckList": Key Down {
        # "Update symbols on the listbox\nLeft and right keys check and uncheck"
        n271 = event-data() -> ("VKey"=w425:T22)  [unwired: 1 in]
        n272 = case shown="\"Left\", \"Right\"" w425 {
          selector: w425 -> [w430 _]
          tunnel: eventvkey."Left" ("VKey") -> [w428 _]
          frame "Left", "Right" {
            n273 = Equal?(x=w428, y=w430) -> (x = y?=w429:bool)
            n274 = Select(t=0, s=w429, f=1) -> (s? t:f=w431:i32)
            n275 = property on="CheckList" class="LstBox (strict)"() -> ("Item Symbols"=w434:i32[])  [unwired: 2 in, 2 out]
            n276 = Replace Array Subset(array=w434, new element=w431, index="CheckList") -> (w433:i32[])
            n277 = property on="CheckList" class="LstBox (strict)"("Item Symbols"=w433) -> ()  [unwired: 2 in, 2 out]
          }
          frame Default {
          }
        }
      }
      event "Motor.Enable": Value Change {
        # "When the test mode otor enable helper is set, update that\ntree row item's value"
        n278 = event-data() -> ("NewVal"=w440:bool)  [unwired: 1 in]
        n279 = Unbundle("Motor") -> ("Value"=w439:dbl)  [unwired: 1 out]
        n280 = Select(t=w439, s=w440, f=0.0) -> (s? t:f=w437:dbl)
        n281 = call <vilib>:"NT Write Number.vi"("Numeric"=w437, "Name"=w436) -> ()  [unwired: 9 in, 1 out]
      }
      event "Test Slider": Value Change {
        # "When the test mode slider helper is set, update that\ntree row item's value"
        n282 = event-data() -> ("NewVal"=w443:dbl)  [unwired: 1 in]
        n283 = call <vilib>:"NT Write Number.vi"("Numeric"=w443, "Name"=w444) -> ()  [unwired: 9 in, 1 out]
      }
      event "On/Off": Value Change {
        # "When the test mode on/off helper value is set, update that\ntree row item's value"
        n284 = event-data() -> ("NewVal"=w448:bool)  [unwired: 1 in]
        n285 = Boolean To (0,1)(Boolean=w448) -> (0, 1=w447:i16)
        n286 = call <vilib>:"NT Write Number.vi"("Numeric"=w447, "Name"=w446) -> ()  [unwired: 9 in, 1 out]
      }
      event "Rev/Fwd": Value Change {
        # "When the test mode helper value for relays is set, update that\ntree row item's value"
        n287 = event-data() -> ("NewVal.Forward"=w456:bool, "NewVal.Reverse"=w455:bool)  [unwired: 1 in]
        n288 = Boolean To (0,1)(Boolean=w456) -> (0, 1=w452:i16)
        n289 = Boolean To (0,1)(Boolean=w455) -> (0, 1=w454:i16)
        n290 = Negate(x=w454) -> (-x=w453:i16)
        n291 = Add(x=w452, y=w453) -> (x+y=w451:i16)
        n292 = call <vilib>:"NT Write Number.vi"("Numeric"=w451, "Name"=w450) -> ()  [unwired: 9 in, 1 out]
      }
      event "Test Ring": Value Change {
        # "When a test mode helper value is selected from the ring,\nset the tree item's variable to the string value"
        n293 = event-data() -> ("NewVal"=w460:u16)  [unwired: 1 in]
        n294 = property on="Test Ring" class="Ring (strict)"() -> ("Strings []"=w461:string[])  [unwired: 2 in, 2 out]
        n295 = Index Array(array=w461, index=w460) -> (element=w459:string)
        n296 = call <vilib>:"NT Write String.vi"("String"=w459, "Name"=w458) -> ()  [unwired: 9 in, 1 out]
      }
      event "Rec Mode": Value Change {
        # "Update globals for recording mode and path to read log from.\nClear when logging and let NetworkTables set path for vision to\nuse."
        n297 = event-data() -> ("NewVal"=w472:enum32{"Stop", "Record", "Playback"})  [unwired: 1 in]
        n298 = global write "WPI_DashboardLogging Global.vi" "Logging Filename"(path "") -> ()
        n299 = global write "WPI_DashboardLogging Global.vi" "Recording"(w472) -> ()
        n300 = case shown="\"Playback\"" w472 {
          tunnel: w471 -> [_ w474 w483]
          tunnel: [_ _ w482] -> w469
          tunnel: [_ _ w481] -> _
          tunnel: w467 -> [_ _ w479]
          tunnel: cluster{i32, i32} {-250, 170} -> [_ _ w478]
          tunnel: [_ _ T23 {"Image Size"=TRUE, "Image Type"=TRUE, "Pixel Value"=TRUE, "ROI Information"=TRUE, "Zoom Factor"=FALSE} ("Image Information Shown:All Elements")] -> w462
          tunnel: [_ _ TRUE ("Zoom Factor")] -> w463
          tunnel: w465 -> [_ _ w475]
          frame Default {
          }
          frame "Stop", "Record" {
            # "Place Window too"
            n301 = invoke class="VI" method="FP.Close"(reference=w474) -> (reference out=w473:refnum<vi>)  [unwired: 2 in, 2 out]
            n302 = invoke class="VI" method="Abort VI"(reference=w473) -> ()  [unwired: 2 in, 3 out]
          }
          frame "Playback" {
            n303 = call "Open Playback Panel.vi"("Offset"=w478, "DB VI Ref"=w479, "Playback in"=w483) -> ("Playback out"=w480:refnum<vi>)  [unwired: 8 in]
            n304 = register-events(w480, w475) -> (reference out=w482:refnum<event-registration>, error out=w481:errorcluster)  [unwired: 2 in]
          }
        }
        n305 = property on="Camera Image Right" class="ImageControl"("Image Information Shown"=w462, "Image Information Visible"=w463) -> ()  [unwired: 2 in, 2 out]
        n306 = property on="Camera Image" class="ImageControl"("Image Information Shown"=w462, "Image Information Visible"=w463) -> ()  [unwired: 2 in, 2 out]
        n307 = call <vilib>:"WPI_DashboardNT Log FieldName Cache.vi"("Operation"=enum16{"Lookup/Add", "Index", "Clear"}."Clear") -> ()  [unwired: 8 in, 3 out]
      }
      event Panel Close {
        w485 = enum32{"Stop", "Record", "Playback"}."Stop" ("Rec Mode")
        # "Playback window has been closed, abort"
        n308 = event-data() -> ()  [unwired: 1 in, 4 out]
        n309 = local write "Rec Mode"(w485) -> ()
        n310 = global write "WPI_DashboardLogging Global.vi" "Recording"(w485) -> ()
      }
      event Panel Close {
        # "Abort playback window and ourself"
        n311 = event-data() -> ()  [unwired: 1 in, 4 out]
        n312 = invoke class="VI" method="FP.Close"(reference=w489) -> (reference out=w488:refnum<vi>)  [unwired: 2 in, 2 out]
        n313 = invoke class="VI" method="Abort VI"(reference=w488) -> (error out=w487:errorcluster)  [unwired: 2 in, 2 out]
        n314 = invoke class="VI" method="Abort VI"(error in=w487) -> ()  [unwired: 2 in, 3 out]
      }
      event User Event {
        n315 = event-data() -> ("IDs"=w496:cluster{"RPC field ID":u16, "Unique ID":u16}, "String"=w495:string)  [unwired: 1 in]
        n316 = Bundle("IDs"=w496, "String"=w495) -> (w494:T9)  [unwired: 1 in]
        n317 = call <vilib>:"Retrieve RPC Response.vi"("RPC Response"=w494) -> ("Output"=w492:string[][])  [unwired: 10 in]
        n318 = Build Array (concatenate)(w490, w492) -> (w491:string[][])
        n319 = local write "Command Params"(w491) -> ()
        n320 = local write "Cmd Status"("" ("Cmd Status")) -> ()
      }
      event "Tree": Double Click {
        n321 = event-data() -> ("PlatMods"=w502:T26, "Tag"=w499:string)  [unwired: 1 in]
        n322 = Unbundle(w502) -> ("Shift"=w501:bool)  [unwired: 4 out]
        n323 = String Subset(string=w499, length (rest)=1 ("length (rest)")) -> (substring=w498:string)  [unwired: 1 in]
        n324 = Not(x=w501) -> (.not. x?=w500:bool)
        n325 = case shown="\"/\"" w498 {
          tunnel: w499 -> [_ w505]
          tunnel: w500 -> [_ w504]
          frame Default {
          }
          frame "/" {
            n326 = call <vilib>:"NT Update Persistence.vi"("Persistence"=w504, "Name"=w505) -> ()  [unwired: 9 in, 1 out]
          }
        }
      }
    }
  }
  n327 = while {
    tunnel: w65 -> [w507]
    i -> [w510]
    stop <- FALSE stop-if-true
    n328 = Wait (ms)(milliseconds to wait=u32 100) -> ()  [unwired: 1 out]
    n329 = case shown="\"Playback\"" "Rec Mode" {
      tunnel: w510 -> [_ _ w525]
      tunnel: [u32 2829099 ("Base Color") u32 11141120 ("Target Color") w514] -> w506
      frame "Stop", Default {
        # "Reset the color, extra updates don't cost much"
      }
      frame "Record" {
      }
      frame "Playback" {
        # "Playback"
        n330 = Quotient & Remainder(x=w525, y=u32 50 ("milliseconds to wait")) -> (x-y*floor(x/y)=w521:u32)  [unwired: 1 out]
        n331 = Divide(x=w521, y=u32 50 ("milliseconds to wait")) -> (x/y=w518:dbl)
        n332 = Multiply(x=6.283185307179586, y=w518) -> (x*y=w523:dbl)
        n333 = Sine(x=w523) -> (sin(x)=w522:dbl)
        n334 = Absolute Value(x=w522) -> (abs(x)=w515:dbl)
        n335 = call "Interpolate RGB Color.vi"("Proportion"=w515, "Target Color"=u32 30976, "Base Color"=u32 2829099) -> ("Result Color"=w514:u32)  [unwired: 8 in]
      }
    }
    n336 = property class="Pane"(reference=w507, "PaneColor"=w506) -> ()  [unwired: 1 in, 2 out]
  }
  n337 = local write "Dashboard Tab"(T2."Drive" ("Dashboard Tab")) -> ()
  n338 = property on="On/Off" class="Bool (strict)"("Visible"=w36) -> ()  [unwired: 2 in, 2 out]
  n339 = property on="Motor" class="Clust (strict)"("Visible"=w36) -> ()  [unwired: 2 in, 2 out]
  n340 = property on="Progress" class="Clust (strict)"("Visible"=w36) -> ()  [unwired: 2 in, 2 out]
  n341 = property on="Test Ring" class="Ring (strict)"("Visible"=w36) -> ()  [unwired: 2 in, 2 out]
  n342 = property on="Rev/Fwd" class="Clust (strict)"("Visible"=w36) -> ()  [unwired: 2 in, 2 out]
  n343 = while {
    tunnel: u16 1741 ("timeout ms (25000)") -> [w527]
    stop <- FALSE stop-if-true
    n344 = TCP Create Listener(10:w527) -> (0:w526:errorcluster, 3:w528:refnum<k5>)  [unwired: 4 in, 1 out]
    n345 = case shown="No Error" w526 {
      selector: w526 -> [w530 _]
      tunnel: w528 -> [w531 _]
      frame No Error {
        n346 = while {
          tunnel: w531 -> [w534]
          tunnel: w530 -> [w533]
          stop <- FALSE stop-if-true
          n347 = TCP Wait On Listener(8:w533, 11:w534) -> (0:w535:errorcluster, 4:w536:refnum<k5>)  [unwired: 2 in, 3 out]
          n348 = local write "TCP"(w536) -> ()
          n349 = case shown="No Error" w535 {
            frame No Error {
            }
            frame Error {
              n350 = Wait (ms)(milliseconds to wait=u32 1000) -> ()  [unwired: 1 out]
            }
          }
        }
      }
      frame Error {
        n351 = Wait (ms)(milliseconds to wait=u32 1000) -> ()  [unwired: 1 out]
      }
    }
  }
  n352 = local write "Command Selection"(u16 0 ("milliseconds to wait")) -> ()
  n353 = local write "Command Params"(string[][] [] ("Command Params")) -> ()
  n354 = global write "WPI_DashboardLogging Global.vi" "Recording"(w59) -> ()
  n355 = local write "Rec Mode"(w59) -> ()
  n356 = call <vilib>:"NT Write String.vi"("String"="Select Auto", "Name"="Auto Selector") -> ()  [unwired: 9 in, 1 out]
